vi "W to kw.vi"(10 "kw?":bool, 11 "P[W]":dbl) -> (3 "P3 out":dbl)   [LabVIEW 2019]
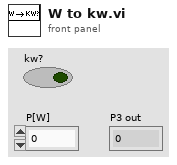
[diagram p1: front panel]
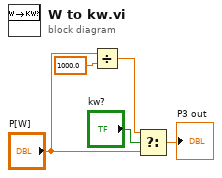
[diagram p0: block diagram]
diagram:
  n1 = Divide(x="P[W]", y=1000.0) -> (x/y=w3:dbl)
  n2 = Select(t=w3, s="kw?", f="P[W]") -> (s? t:f=→"P3 out":dbl)
